vi "AMZ_S3_Create String to Sign.vi"(6 "HTTP-Verb":string(combo)="GET", 8 "error in (no error)":errorcluster, 9 "Bucket in":string, 10 "Path and query string":string, 11 "HTTP Headers in":T1[](array[typedef])) -> (0 "error out":errorcluster, 2 "StringToSign":string, 3 "HTTP Headers":T1[](array[typedef]))   [LabVIEW 2015, in "LV Interface for Amazon S3.lvlib"]
doc: "Create the String to Sign. It will be used as the Authorization header after it is signed with the SecretKey."
uses:
  LV Interface for Amazon S3.lvlib
  Typedefs/AMZ_S3_HTTP Header-Value pair.ctl
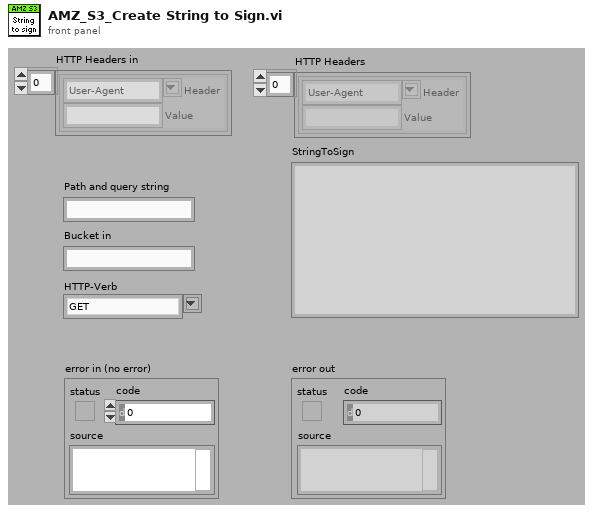
[diagram p1: front panel]
types:
  T1 = typedef "LV Interface for Amazon S3.lvlib/AMZ_S3_HTTP Header-Value pair.ctl" = cluster{"Header":string, "Value":string}
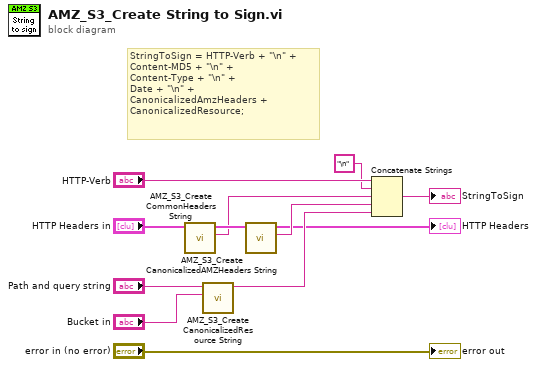
[diagram p0: block diagram]
diagram:
  # "StringToSign = HTTP-Verb + \"\\n\" +\nContent-MD5 + \"\\n\" +\nContent-Type + \"\\n\" +\nDate + \"\\n\" +\nCanonicalizedAmzHeaders +\nCanonicalizedResource;"
  n1 = call "AMZ_S3_Create CommonHeaders String.vi"("HTTP Headers in"="HTTP Headers in") -> ("CommonHeaderValues"=w5:string, "HTTP Headers"=w12:T1[])  [unwired: 9 in]
  n2 = call "AMZ_S3_Create CanonicalizedResource String.vi"("Bucket"="Bucket in", "Path and query string"="Path and query string") -> ("Canonicalized Resource"=w6:string)  [unwired: 9 in]
  n3 = call "AMZ_S3_Create CanonicalizedAMZHeaders String.vi"("HTTP Headers in"=w12) -> ("CanonicalizedAMZHeaders"=w4:string, "HTTP Headers"=→"HTTP Headers":T1[])  [unwired: 9 in]
  n4 = Concatenate Strings("HTTP-Verb", "\n", w5, w4, w6) -> (→"StringToSign":string)
  "error out" <- "error in (no error)"
